vi "Timeout.vi"(8 "error in (no error)":errorcluster, 10 "Data":variant, 11 "Log in":refnum<class "Log.lvclass">) -> (0 "error out":errorcluster, 3 "Log out":refnum<class "Log.lvclass">)   [LabVIEW 2015, in "AMS UI.lvlib" / "Log.lvclass"]
uses:
  Log.lvclass
  AMS Gas Actor/AMS Gas Actor.lvclass
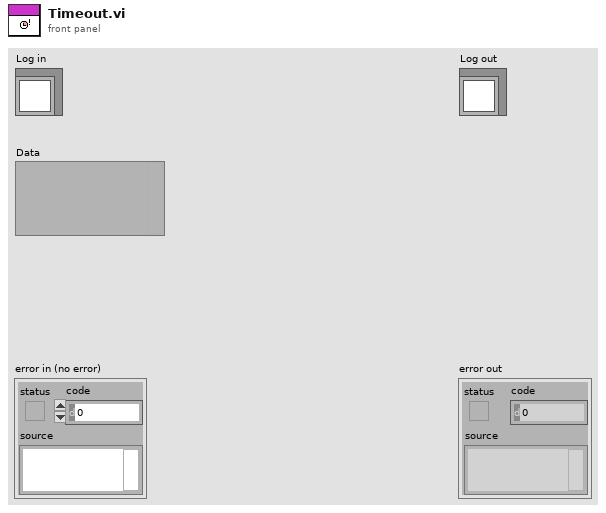
[diagram p1: front panel]
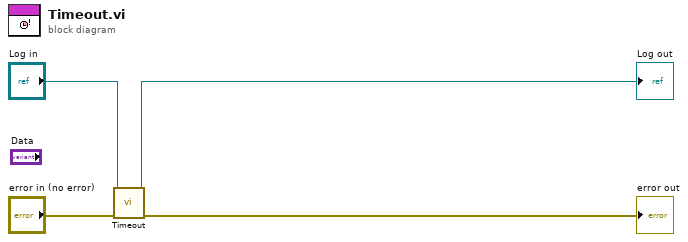
[diagram p0: block diagram]
diagram:
  n1 = call-parent "Timeout.vi"("error in (no error)"="error in (no error)", "eActor in"="Log in") -> ("error out"=→"error out":errorcluster, "eActor out"=→"Log out":refnum<class "Log.lvclass">)  [unwired: 8 in]
